vi "FGV Algebraic.vi"(6 "Aktionen Algebraic":T1, 7 "Istwerte":sgl[](array[numeric]), 9 "Variablen":string[](array[string]), 10 "Formel":string[](array[string]), 11 "Namen":string[](array[string])) -> (1 "Variablen":string[](array[string]), 2 "Formel":string[](array[string]), 3 "Namen":string[](array[string]), 4 "Rohwerte":sgl[](array[numeric]), 5 "Messdaten":sgl[](array[numeric]))   [LabVIEW 2020, in "FT-IR.lvlib" / "Algebraic Modul.lvlib"]
uses:
  Algebraic Modul.lvlib
  FGV Algebraic Aktionen.ctl
  Allgemein/allgemeine Sub-VIs.lvlib
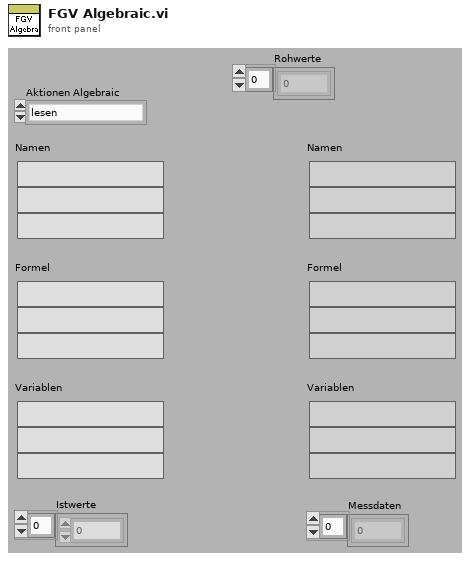
[diagram p1: front panel]
types:
  T1 = typedef "FT-IR.lvlib/Algebraic Modul.lvlib/FGV Algebraic Aktionen.ctl" = enum16{"lesen", "laden", "speichern", "berechnen", "schreiben"}
  T2 = cluster{"Namen":string[], "Formel":string[], "Variablen":string[]}
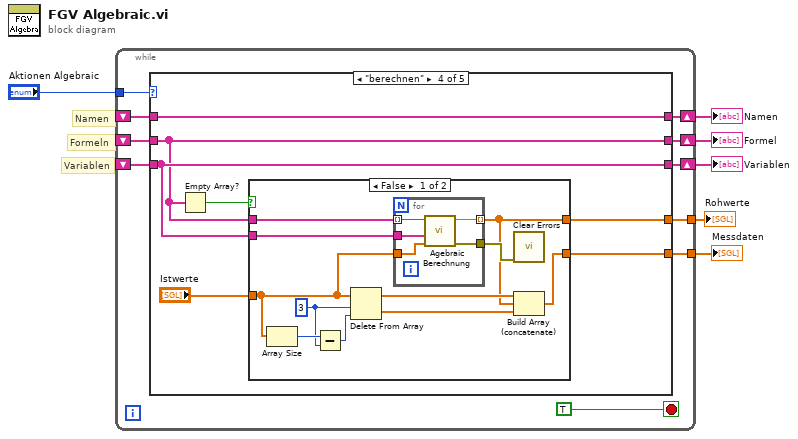
[diagram p0: block diagram]
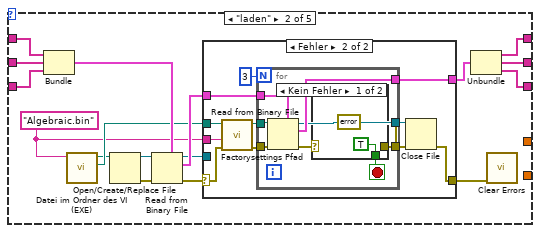
[diagram p3: hidden frame]
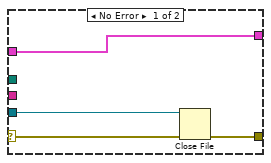
[diagram p4: hidden frame]
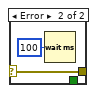
[diagram p5: hidden frame]
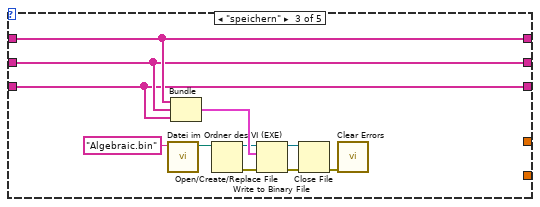
[diagram p6: hidden frame]
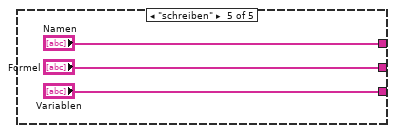
[diagram p8: hidden frame]
diagram:
  # "Variablen"
  # "Formeln"
  # "Namen"
  n1 = while {
    tunnel: "Aktionen Algebraic" -> [w15]
    shift-right: [w14] -> w5
    shift-left: _ -> [w11]
    shift-right: [w13] -> w4
    shift-left: _ -> [w10]
    shift-right: [w12] -> w3
    shift-left: _ -> [w9]
    tunnel: [w8] -> w2
    tunnel: [w7] -> w1
    stop <- TRUE stop-if-true
    n2 = case shown="\"berechnen\"" w15 {
      tunnel: [w19 w32 w73 w81 "Namen"] -> w14
      tunnel: [w18 w31 w72 w76 "Formel"] -> w13
      tunnel: [w17 w30 w71 w80 "Variablen"] -> w12
      tunnel: w11 -> [w19 w36 w73 w81 _]
      tunnel: w10 -> [w18 w35 w72 w76 _]
      tunnel: w9 -> [w17 w34 w71 w80 _]
      tunnel: [_ _ _ w78 _] -> w8
      tunnel: [_ _ _ w75 _] -> w7
      frame "lesen", Default {
      }
      frame "laden" {
        w25 = "Algebraic.bin" ("Dateiname")
        n3 = Bundle("Namen"=w36, "Formel"=w35, "Variablen"=w34) -> (w33:T2)  [unwired: 1 in]
        n4 = call "Datei im Ordner des VI (EXE).vi"("Dateiname"=w25) -> ("Ordner des Haupt-VIs"=w26:path, "Dateipfad im Ordner des Haupt-VIs"=w22:path)  [unwired: 8 in, 1 out]
        n5 = Open/Create/Replace File(file path (use dialog)=w22) -> (refnum out=w21:refnum<file>, error out=w20:errorcluster)  [unwired: 5 in, 1 out]
        n6 = Read from Binary File(5:w33, 8:w20, 11:w21) -> (0:w29:errorcluster, 2:w28:T2, 3:w27:refnum<file>)  [unwired: 4 out]
        n7 = case shown="Fehler" w29 {
          selector: w29 -> [w39 w43]
          tunnel: w26 -> [_ w44]
          tunnel: w28 -> [w40 w42]
          tunnel: [w40 w50] -> w23
          tunnel: [w37 w48] -> w24
          tunnel: w27 -> [w38 _]
          tunnel: w25 -> [_ w41]
          frame No Error {
            n8 = Close File(refnum=w38, error in=w39) -> (error out=w37:errorcluster)  [unwired: 1 out]
          }
          frame Error {
            n9 = call "Factorysettings Pfad.vi"("error in (no error)"=w43, "Dateiname"=w41, "Ordner des Haupt-VIs"=w44) -> ("error out"=w45:errorcluster, "Pfad Factorysettings"=w46:path)  [unwired: 7 in]
            n10 = for {
              N: 3 -> [_]
              tunnel: w45 -> [w57]
              tunnel: w46 -> [w56]
              tunnel: [w55] -> w50
              tunnel: [w54] -> w49
              tunnel: [w53] -> w47
              tunnel: w42 -> [w52]
              stop <- w58 stop-if-true
              n11 = Read from Binary File(5:w52, 8:w57, 11:w56) -> (0:w59:errorcluster, 2:w55:T2, 3:w53:refnum<file>)  [unwired: 3 in, 1 out]
              n12 = case shown="Kein Fehler" w59 {
                selector: w59 -> [_ w62]
                tunnel: [TRUE _] -> w58
                tunnel: [errorcluster {"status"=FALSE, "code"=0, "source"=""} ("error IO") w62] -> w54
                frame No Error {
                }
                frame Error {
                  n13 = Wait (ms)(milliseconds to wait=u32 100 ("Zu wartende ms")) -> ()  [unwired: 1 out]
                }
              }
            }
            n14 = Close File(refnum=w47, error in=w49) -> (error out=w48:errorcluster)  [unwired: 1 out]
          }
        }
        n15 = Unbundle(w23) -> ("Namen"=w32:string[], "Formel"=w31:string[], "Variablen"=w30:string[])
        n16 = call <vilib>:"Clear Errors.vi"("error in (no error)"=w24) -> ()  [unwired: 5 in, 2 out]
      }
      frame "speichern" {
        n17 = call "Datei im Ordner des VI (EXE).vi"("Dateiname"="Algebraic.bin") -> ("Dateipfad im Ordner des Haupt-VIs"=w68:path)  [unwired: 8 in, 2 out]
        n18 = Bundle("Namen"=w73, "Formel"=w72, "Variablen"=w71) -> (w70:T2)  [unwired: 1 in]
        n19 = Open/Create/Replace File(file path (use dialog)=w68) -> (refnum out=w67:refnum<file>, error out=w69:errorcluster)  [unwired: 5 in, 1 out]
        n20 = Write to Binary File(file (use dialog)=w67, data=w70, error in=w69) -> (refnum out=w65:refnum<file>, error out=w66:errorcluster)  [unwired: 4 out]
        n21 = Close File(refnum=w65, error in=w66) -> (error out=w64:errorcluster)  [unwired: 1 out]
        n22 = call <vilib>:"Clear Errors.vi"("error in (no error)"=w64) -> ()  [unwired: 5 in, 2 out]
      }
      frame "berechnen" {
        n23 = Empty Array?(array=w76) -> (empty?=w77:bool)
        n24 = case shown="False" w77 {
          tunnel: w80 -> [w91 _]
          tunnel: w76 -> [w90 _]
          tunnel: "Istwerte" -> [w83 w98]
          tunnel: [w89 w98] -> w78
          tunnel: [w82 _] -> w75
          frame False {
            w84 = 3 ("Länge")
            n25 = Array Size(array=w83) -> (size(s)=w86:i32)
            n26 = Subtract(x=w86, y=w84) -> (x-y=w85:i32)
            n27 = Delete From Array(array=w83, length=w84, index=w85) -> (deleted portion=w87:sgl[], array with subset deleted=w88:sgl[])
            n28 = for {
              tunnel: w91 -> [w97]
              tunnel: w90 -> [w96] mode=indexing
              tunnel: [w95] -> w82 mode=indexing
              tunnel: w83 -> [w94]
              tunnel: [w93] -> w92
              n29 = call "Agebraic Berechnung.vi"("X Values"=w94, "Variables"=w97, "formula"=w96) -> ("error out"=w93:errorcluster, "y value"=w95:sgl)  [unwired: 7 in]
            }
            n30 = call <vilib>:"Clear Errors.vi"("error in (no error)"=w92) -> ()  [unwired: 5 in, 2 out]
            n31 = Build Array (concatenate)(w88, w82, w87) -> (w89:sgl[])
          }
          frame True {
          }
        }
      }
      frame "schreiben" {
      }
    }
  }
  "Variablen" <- w3
  "Namen" <- w5
  "Formel" <- w4
  "Messdaten" <- w2
  "Rohwerte" <- w1
